vi "Load Target.vi"(8 "error in":errorcluster, 10 "Target String":string, 11 "Sentence in":refnum<class "Sentence.lvclass">) -> (0 "error out":errorcluster, 3 "Sentence out":refnum<class "Sentence.lvclass">)   [LabVIEW 2016, in "Sentence.lvclass"]
uses:
  Sentence.lvclass
  Gene/Character.lvclass
  IChromosome/IChromosome.lvclass
  C:/Users/J51654/My Projects/Evolutionary Programming/GA Framework/IGene/IGene.lvclass
  C:/Users/J51654/My Projects/Evolutionary Programming/GA Framework/IChromosome/IChromosome.lvclass
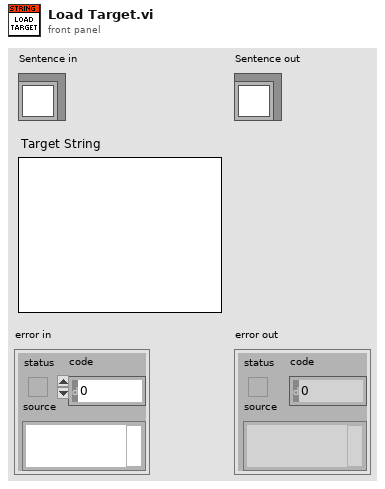
[diagram p1: front panel]
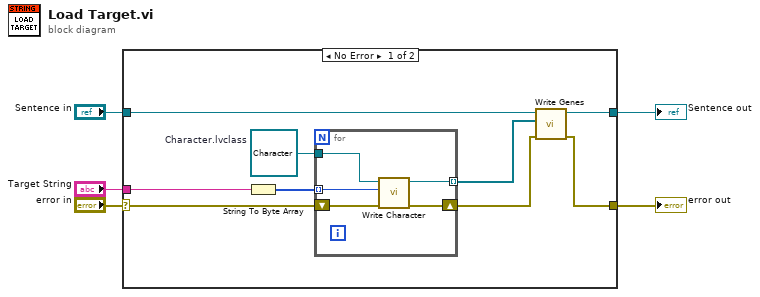
[diagram p0: block diagram]
diagram:
  n1 = case shown="No Error" "error in" {
    selector: "error in" -> [w11 w21]
    tunnel: [w6 w21] -> w4
    tunnel: [w9 w20] -> w2
    tunnel: "Sentence in" -> [w10 w20]
    tunnel: "Target String" -> [w13 _]
    frame No Error {
      w14 = refnum<class "Character.lvclass"> refnum  # Character.lvclass
      n2 = String To Byte Array(string=w13) -> (unsigned byte array=w12:u8[])
      n3 = for {
        tunnel: w14 -> [w19]
        tunnel: w12 -> [w18] mode=indexing
        tunnel: [w17] -> w8 mode=indexing
        shift-right: [w15] -> w7
        shift-left: w11 -> [w16]
        n4 = call "Write Character.vi"("error in (no error)"=w16, "Character"=w18, "Character in"=w19) -> ("error out"=w15:errorcluster, "Character out"=w17:refnum<class "Character.lvclass">)  [unwired: 7 in]
      }
      n5 = call "Write Genes.vi"("error in"=w7, "Genes"=w8, "IChromosome in"=w10) -> ("error out"=w6:errorcluster, "IChromosome out"=w9:refnum<class "Sentence.lvclass">)  [unwired: 7 in]
    }
    frame Error {
    }
  }
  "error out" <- w4
  "Sentence out" <- w2
